vi "Convert to Action Data (JSON).vi"(1 "Data Types":T1(array[cluster]), 2 "Data Names&Data":string[][](array[string])) -> (0 "Action Data (JSON)":string)   [LabVIEW 2016, in "Hardware.lvlib" / "Motions.lvlib" / "Motions.lvclass"]
uses:
  <userlib>/Common Components/Hardware/Abstract System/Motions/Motions/Motions.lvclass
  <vilib>/addons/JSON API/JSON Object/Set Object Item by name.vi
  <vilib>/addons/JSON API/JSON Scalar/JSON Scalar.lvclass
  C:/Program Files (x86)/National Instruments/LabVIEW 2016/vi.lib/addons/JSON API/JSON Value/JSON Value.lvclass
  <vilib>/addons/JSON API/JSON Object/JSON Object.lvclass
  <vilib>/addons/JSON API/JSON Scalar/Set I32.vi
  <vilib>/addons/JSON API/JSON Scalar/Set DBL.vi
  <vilib>/addons/JSON API/JSON Scalar/Set Boolean.vi
  <vilib>/addons/JSON API/JSON Scalar/Set String.vi
  <vilib>/addons/JSON API/JSON Value/Get as JSON string (pretty).vi
  <vilib>/addons/JSON API/Get Polymorphic/JSON GetSet.lvlib
  <vilib>/addons/JSON API/JSON Value/JSON Value.lvclass
panel:
  # "Index is converted to Motor"
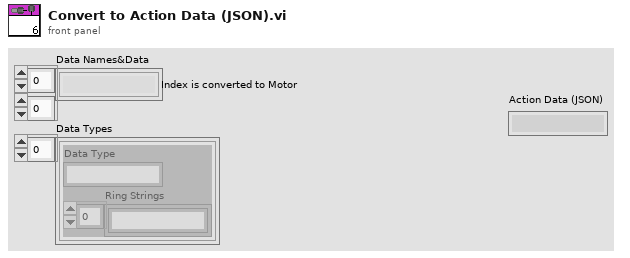
[diagram p1: front panel]
types:
  T1 = cluster{"Data Type":string, "Ring Strings":string[]}[]
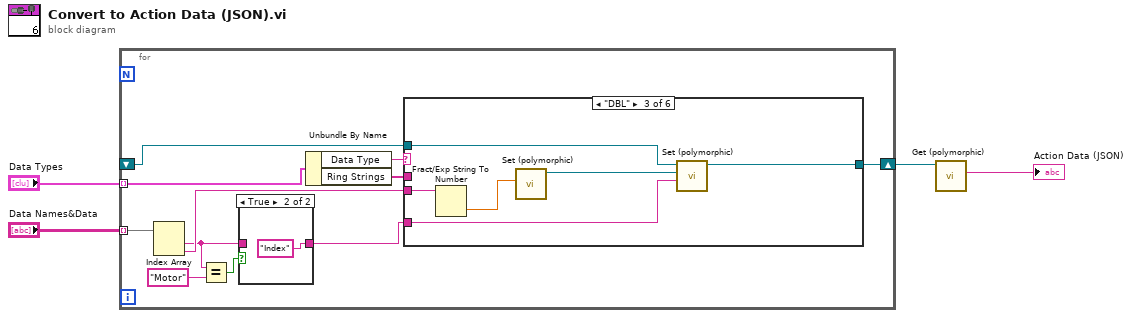
[diagram p0: block diagram]
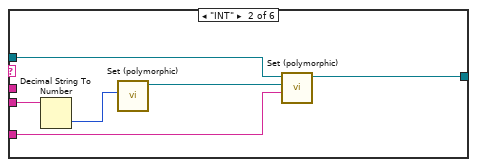
[diagram p4: hidden frame]
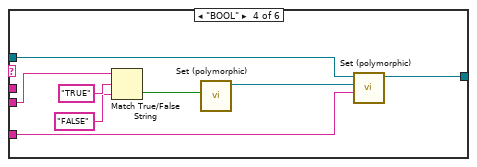
[diagram p5: hidden frame]
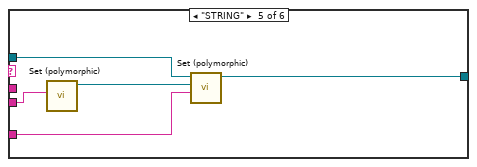
[diagram p6: hidden frame]
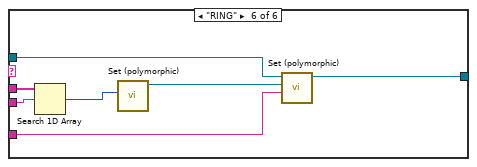
[diagram p7: hidden frame]
diagram:
  n1 = for {
    tunnel: "Data Names&Data" -> [w15] mode=indexing
    tunnel: "Data Types" -> [w14] mode=indexing
    shift-right: [w11] -> w2
    shift-left: _ -> [w10]
    n2 = Index Array(array=w15) -> (element #1=w7:string, element #2=w12:string)  [unwired: 2 in]
    n3 = Equal?(x=w7, y="Motor") -> (x = y?=w8:bool)
    n4 = case shown="True" w8 {
      tunnel: w7 -> [w16 _]
      tunnel: [w16 "Index" ("y")] -> w6
      frame False {
      }
      frame True {
      }
    }
    n5 = Unbundle By Name(w14) -> ("Data Type"=w13:string, "Ring Strings"=w5:string[])
    n6 = case shown="\"DBL\"" w13 {
      tunnel: w12 -> [_ w24 w30 w38 w39 w45]
      tunnel: w6 -> [_ w21 w27 w35 w42 w49]
      tunnel: [w18 w20 w26 w34 w41 w48] -> w11
      tunnel: w10 -> [w18 w19 w25 w33 w40 w47]
      tunnel: w5 -> [_ _ _ _ _ w46]
      frame Default {
      }
      frame "INT" {
        n7 = Decimal String To Number(string=w24) -> (number=w23:i32)  [unwired: 2 in, 1 out]
        n8 = call-poly <vilib>:"Set (polymorphic).vi"("Numeric"=w23) -> ("JSON Scalar out"=w22:refnum<class "JSON Scalar.lvclass">)  [unwired: 9 in, 1 out]
        n9 = call-poly <vilib>:"Set (polymorphic).vi"("name"=w21, "Value"=w22, "JSON Object in"=w19) -> ("JSON Object out"=w20:refnum<class "JSON Object.lvclass">)  [unwired: 6 in, 2 out]
      }
      frame "DBL" {
        n10 = Fract/Exp String To Number(string=w30) -> (number=w29:dbl)  [unwired: 3 in, 1 out]
        n11 = call-poly <vilib>:"Set (polymorphic).vi"("Numeric"=w29) -> ("JSON Scalar out"=w28:refnum<class "JSON Scalar.lvclass">)  [unwired: 9 in, 1 out]
        n12 = call-poly <vilib>:"Set (polymorphic).vi"("name"=w27, "Value"=w28, "JSON Object in"=w25) -> ("JSON Object out"=w26:refnum<class "JSON Object.lvclass">)  [unwired: 6 in, 2 out]
      }
      frame "BOOL" {
        n13 = Match True/False String(2:"FALSE" ("false string"), 3:"TRUE" ("true string"), 4:w38) -> (0:w37:bool)  [unwired: 1 out]
        n14 = call-poly <vilib>:"Set (polymorphic).vi"("Boolean"=w37) -> ("JSON Scalar out"=w36:refnum<class "JSON Scalar.lvclass">)  [unwired: 9 in, 1 out]
        n15 = call-poly <vilib>:"Set (polymorphic).vi"("name"=w35, "Value"=w36, "JSON Object in"=w33) -> ("JSON Object out"=w34:refnum<class "JSON Object.lvclass">)  [unwired: 6 in, 2 out]
      }
      frame "STRING" {
        n16 = call-poly <vilib>:"Set (polymorphic).vi"("String"=w39) -> ("JSON Scalar out"=w43:refnum<class "JSON Scalar.lvclass">)  [unwired: 9 in, 1 out]
        n17 = call-poly <vilib>:"Set (polymorphic).vi"("name"=w42, "Value"=w43, "JSON Object in"=w40) -> ("JSON Object out"=w41:refnum<class "JSON Object.lvclass">)  [unwired: 6 in, 2 out]
      }
      frame "RING" {
        n18 = Search 1D Array(1D array=w46, element=w45) -> (index of element=w44:i32)  [unwired: 1 in]
        n19 = call-poly <vilib>:"Set (polymorphic).vi"("Numeric"=w44) -> ("JSON Scalar out"=w50:refnum<class "JSON Scalar.lvclass">)  [unwired: 9 in, 1 out]
        n20 = call-poly <vilib>:"Set (polymorphic).vi"("name"=w49, "Value"=w50, "JSON Object in"=w47) -> ("JSON Object out"=w48:refnum<class "JSON Object.lvclass">)  [unwired: 6 in, 2 out]
      }
    }
  }
  n21 = call-poly <vilib>:"Get (polymorphic).vi"("JSON Value in"=w2) -> ("<JSON>"=→"Action Data (JSON)":string)  [unwired: 9 in, 1 out]
